vi "CAN Position Control Encoder.vi"() -> ()   [LabVIEW 2014]
doc: "This example shows how to position a motor using CAN Jaguar and a quadrature encoder. For details setting up and understanding CAN Jaguar, see the Can Jaguar Fundamentals tutorial accessable from the LabVIEW Getting Started Window.\n\nTo position the motor, a PID control loop runs on the Jaguar. Notice that the encoder is wired directly to the Jaguar. One advantage of this is that the PID control does not use resources on the roboRIO. One disadvantage is that the PID code cannot be viewed or changed. However, the control can be tuned by changing the PID Parameters.\n\nOn the diagram, notice that in order to apply new PID tuning parameters, the motor must first be disabled, and then enabled afterward. Also notice that since the control loop runs on the Jaguar, the LabVIEW loop delay is set to a slow 100ms. In fact the only reason this loop needs to run is to send a new set position, read the current position, or apply new tuning parameters.\n\nCorrect tuning parameters for a PID controller are dependent on the complete system of the motor and the load. It will be difficult to tune this system if there is no load attached to the motor. While this example is not a PID tutorial, the following information may help in understanding how to tune your PID control system.\n\nP (proportional) depends on the present error, I (integral) on the accumulation of past errors, and D (derivative) is a prediction of future errors, based on the current rate of change. The proportional parameter (P) will reduce the rise time and will reduce, but never eliminate, the steady-state error. The integral parameter (I) will eliminate the steady-state error, but may make the transient response worse. The derivative parameter (D) will increase the stability of the system, reducing the overshoot, and improving the transient response. The effects of each parameter are summarized in a table on the front panel.\n\nThis example expects a USB cable connected from your development PC to the Type B USB Jack (next to the power input) on the roboRIO.\n\nThis example requires the Driver Station to be running with Teleoperated Enabled."
uses:
  <vilib>/Rock Robotics/WPI/CAN/Jaguar/SubVIs/WPI_CANJaguar_ControlMode.ctl
  <vilib>/Rock Robotics/WPI/CAN/Jaguar/SubVIs/WPI_CANJaguar_PositionReference.ctl
  <vilib>/Rock Robotics/WPI/CAN/Jaguar/SubVIs/WPI_CANJaguar_LimitMode.ctl
  <vilib>/Rock Robotics/WPI/CAN/Jaguar/SubVIs/WPI_CANJaguar_BrakeCoastMode.ctl
  <vilib>/Rock Robotics/WPI/CAN/Jaguar/SubVIs/WPI_CANJaguar_StatusSelect.ctl
  <vilib>/Rock Robotics/WPI/MotorControl/WPI_MotorControlOpenCANJaguar.vi
panel:
  in  "PID Tuning":string[][](table)=[["Parameter", "Rise Time", "Overshoot", "Settling\nTime", "Steady State\nError"], ["P", "decrease", "increase", "small\nchange", "decrease"], ["I", "decrease", "increase", "increase", "eliminate"], ["D", "small\nchange", "decrease", "decrease", "small\nchange"]]
  out "Actual Position (revolutions)":dbl(slide) scale=-10.0..10.0
  in  "D2":dbl=15.0 caption="D"
  in  "I2":dbl=0.005 caption="I"
  in  "P2":dbl=500.0 caption="P"
  in  "apply new PID":bool
  in  "D":dbl=15.0
  in  "I":dbl=0.005
  in  "P":dbl=500.0
  in  "Set Position (revolutions)":dbl(slide) scale=-10.0..10.0
  in  "Maximum Output Voltage":dbl=12.0
  in  "Reverse Limit Position":dbl=-50.0
  in  "Forward Limit Position":dbl=50.0
  in  "Encoder Codes Per Rev":u16=1250
  in  "Device Number":u8=1
  in  "stop":bool
  # "Set these inputs before running."
  # "These can be set while running."
  # "Power\nTerminals"
  # "Motor\nTerminals"
  # "Looking at the RJ12 socket on the Jaguar, standard wire colors are shown for an inserted cable.  CAN only uses pins 3 and 4.\npin 3 (red) = CAN H\npin 4 (green) = CAN L"
  # "To roboRIO CAN terminals"
  # "Terminator plug"
  # "Black Jaguar"
  # "A"
  # "B"
  # "Index"
  # "+5V"
  # "Gnd"
  # "Encoder"
  # "white\nblack\nred\ngreen\nyellow\nblue"
  # "1   2   3   4   5   6"
  # "Runtime Tuning"
  # "PID Parameters"
  # "Initial PID Parameters"
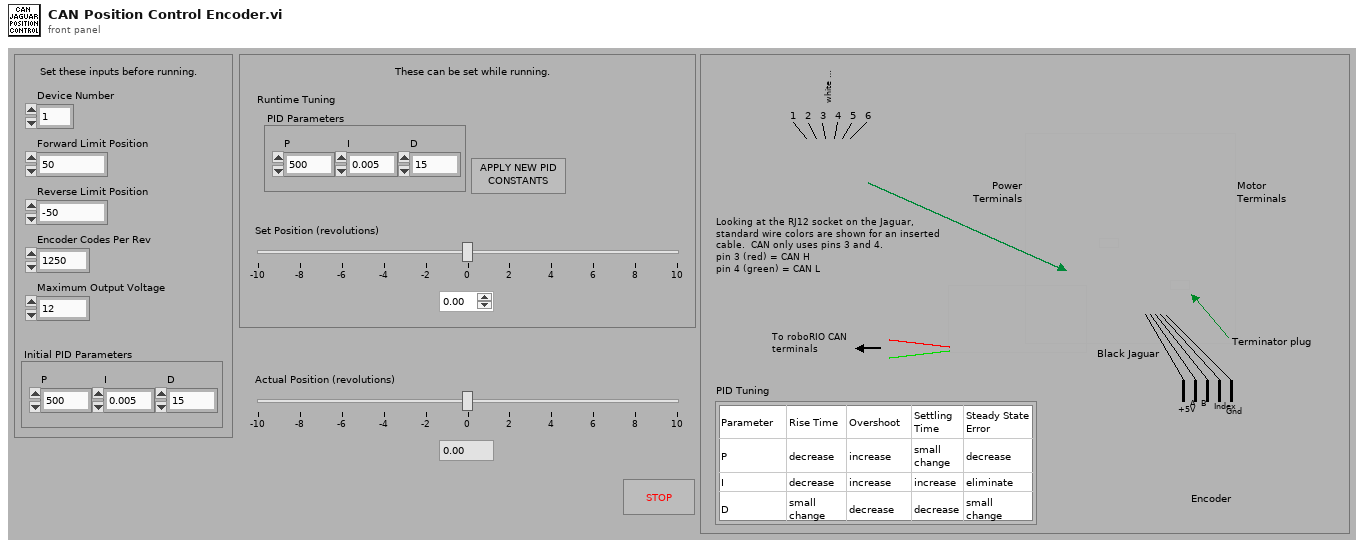
[diagram p1: front panel]
types:
  T1 = typedef "WPI_CANJaguar_StatusSelect.ctl" = enum16{"Output Percent VBus", "Output Voltage", "Bus Voltage", "Current", "Temperature", "Position", "Speed", "Limit Switches", "Faults", "Fault Counters", "Power Cycle"}
  T2 = typedef "WPI_CANJaguar_BrakeCoastMode.ctl" = enum8{"Jumper", "Brake", "Coast"}
  T3 = typedef "WPI_CANJaguar_LimitMode.ctl" = enum16{"Switch Inputs Only", "Soft Position Limits"}
  T4 = typedef "WPI_CANJaguar_PositionReference.ctl" = u8
  T5 = typedef "WPI_CANJaguar_ControlMode.ctl" = enum8{"Percent VBus", "Current", "Speed", "Position", "Voltage"}
  T6 = typedef "WPI_MotorControlDeviceRef.ctl" = cluster{"DeviceStatus":errorcluster, "Type":T7, "PWM":cluster{"Controller":T8, "PWM Channel":T9, "DeadBand":T10}, "CAN":cluster{"Device Number":u8, "Control Mode":T5, "Semaphore":T11, "Max Vout":dbl, "TalonSRX Control Mode":T12}, "Invert":bool, "TransformRef":T13, "InvTransformRef":T13}
  T7 = typedef "WPI_MotorControlType.ctl" = enum16{"PWM", "CAN", "CANTalonSRX"}
  T8 = typedef "FPGA_TypedefDigitalModule.ctl" = enum16{"Controller 1"}
  T9 = typedef "FPGA_DIOPWMChannel.ctl" = enum8{"PWM 0", "PWM 1", "PWM 2", "PWM 3", "PWM 4", "PWM 5", "PWM 6", "PWM 7", "PWM 8", "PWM 9", "PWM MXP 0", "PWM MXP 1", "PWM MXP 2", "PWM MXP 3", "PWM MXP 4", "PWM MXP 5", "PWM MXP 6", "PWM MXP 7", "PWM MXP 8", "PWM MXP 9", "Invalid"}
  T10 = typedef "WPI_PWMDeadband.ctl" = cluster{"Name":string, "maxPositivePwm":i32, "minPositivePwm":i32, "centerPwm":i32, "maxNegativePwm":i32, "minNegativePwm":i32, "angularRange":u16}
  T11 = typedef "Semaphore RefNum" = refnum<k1>
  T12 = typedef "WPI_CANTalonSRX_APIControlMode.ctl" = enum8{"Percent VBus", "Speed", "Position", "Slave", "Unchanged / Invalid"}
  T13 = typedef "WPI_PWMTransform_ConPane.ctl" = refnum<vi>
  T14 = typedef "WPI_CANJaguar_Status.ctl" = cluster{"Output Percent VBus":dbl, "Output Voltage":dbl, "Bus Voltage":dbl, "Current":dbl, "Temperature":dbl, "Position":dbl, "Speed":dbl, "Limits":cluster{"Forward Limit":bool, "Reverse Limit":bool, "Forward Soft Limit":bool, "Reverse Soft Limit":bool, "Sticky Forward Limit":bool, "Sticky Reverse Limit":bool, "Sticky Forward Soft Limit":bool, "Sticky Reverse Soft Limit":bool}, "Faults":cluster{"Current Fault":bool, "Temperature Fault":bool, "Bus Voltage Fault":bool, "Gate Driver Fault":bool, "Comm Fault":bool}, "Fault Counters":cluster{"Current Faults":u8, "Temperature Faults":u8, "Bus Voltage Faults":u8, "Gate Driver Faults":u8, "Comm Faults":u8, "CAN Status":u8, "CAN RX Errors":u8, "CAN TX Errors":u8}, "Power Cycle":bool}
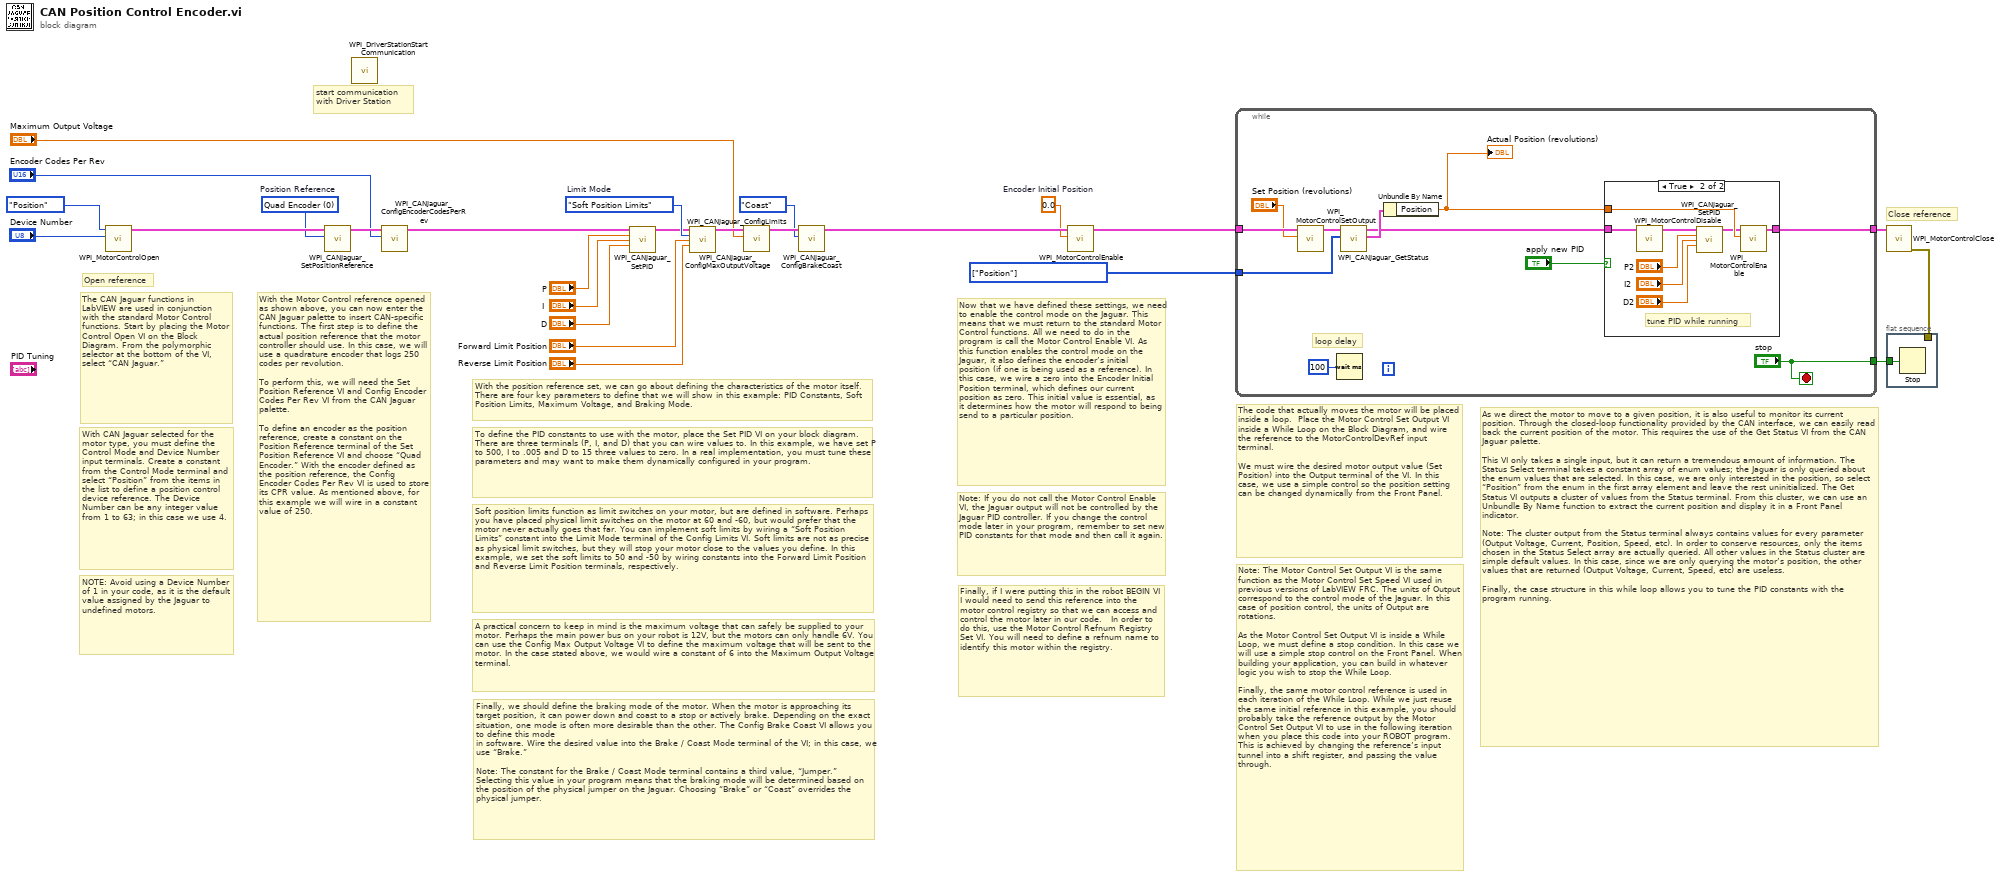
[diagram p0: block diagram]
diagram:
  w6 = 0.0  # Encoder Initial Position
  w7 = T1[] [enum."Position"] items=["Output Percent VBus", "Output Voltage", "Bus Voltage", "Current", "Temperature", "Position", "Speed", "Limit Switches", "Faults", "Fault Counters", "Power Cycle"] ("Status Select")
  w18 = WPI_CANJaguar_LimitMode."Soft Position Limits"  # Limit Mode
  w19 = T4 0 items=["Quad Encoder"=0, "Potentiometer"=1, "None"=255]  # Position Reference
  # "As we direct the motor to move to a given position, it is also useful to monitor its current position. Through the closed-loop functionality provided by the CAN interface, we can easily read back the current position of the motor. This requires the use of the Get Status VI from the CAN Jaguar palette.\n\nThis VI only takes a single input, but it can return a tremendous amount of information. The Status Select terminal takes a constant array of enum values; the Jaguar is only queried about the enum values that are selected. In this case, we are only interested in the position, so select “Position” from the enum in the first array element and leave the rest uninitialized. The Get Status VI outputs a cluster of values from the Status terminal. From this cluster, we can use an Unbundle By Name function to extract the current position and display it in a Front Panel indicator.\n\nNote: The cluster output from the Status terminal always contains values for every parameter (Output Voltage, Current, Position, Speed, etc). In order to conserve resources, only the items chosen in the Status Select array are actually queried. All other values in the Status cluster are simple default values. In this case, since we are only querying the motor’s position, the other values that are returned (Output Voltage, Current, Speed, etc) are useless.\n\nFinally, the case structure in this while loop allows you to tune the PID constants with the program running."
  # "Note: The Motor Control Set Output VI is the same function as the Motor Control Set Speed VI used in previous versions of LabVIEW FRC. The units of Output correspond to the control mode of the Jaguar. In this case of position control, the units of Output are rotations.\n\nAs the Motor Control Set Output VI is inside a While Loop, we must define a stop condition. In this case we will use a simple stop control on the Front Panel. When building your application, you can build in whatever logic you wish to stop the While Loop. \n\nFinally, the same motor control reference is used in each iteration of the While Loop. While we just reuse the same initial reference in this example, you should probably take the reference output by the Motor Control Set Output VI to use in the following iteration when you place this code into your ROBOT program. This is achieved by changing the reference’s input tunnel into a shift register, and passing the value through."
  # "The code that actually moves the motor will be placed inside a loop.  Place the Motor Control Set Output VI inside a While Loop on the Block Diagram, and wire the reference to the MotorControlDevRef input terminal. \n\nWe must wire the desired motor output value (Set Position) into the Output terminal of the VI. In this case, we use a simple control so the position setting can be changed dynamically from the Front Panel."
  # "Finally, if I were putting this in the robot BEGIN VI I would need to send this reference into the motor control registry so that we can access and control the motor later in our code.   In order to do this, use the Motor Control Refnum Registry Set VI. You will need to define a refnum name to identify this motor within the registry."
  # "Note: If you do not call the Motor Control Enable VI, the Jaguar output will not be controlled by the Jaguar PID controller. If you change the control mode later in your program, remember to set new PID constants for that mode and then call it again."
  # "Now that we have defined these settings, we need to enable the control mode on the Jaguar. This means that we must return to the standard Motor Control functions. All we need to do in the program is call the Motor Control Enable VI. As this function enables the control mode on the Jaguar, it also defines the encoder’s initial position (if one is being used as a reference). In this case, we wire a zero into the Encoder Initial Position terminal, which defines our current position as zero. This initial value is essential, as it determines how the motor will respond to being send to a particular position."
  # "Finally, we should define the braking mode of the motor. When the motor is approaching its target position, it can power down and coast to a stop or actively brake. Depending on the exact situation, one mode is often more desirable than the other. The Config Brake Coast VI allows you to define this mode\nin software. Wire the desired value into the Brake / Coast Mode terminal of the VI; in this case, we use “Brake.”\n\nNote: The constant for the Brake / Coast Mode terminal contains a third value, “Jumper.” Selecting this value in your program means that the braking mode will be determined based on the position of the physical jumper on the Jaguar. Choosing “Brake” or “Coast” overrides the physical jumper."
  # "A practical concern to keep in mind is the maximum voltage that can safely be supplied to your motor. Perhaps the main power bus on your robot is 12V, but the motors can only handle 6V. You can use the Config Max Output Voltage VI to define the maximum voltage that will be sent to the motor. In the case stated above, we would wire a constant of 6 into the Maximum Output Voltage terminal."
  # "Soft position limits function as limit switches on your motor, but are defined in software. Perhaps you have placed physical limit switches on the motor at 60 and -60, but would prefer that the motor never actually goes that far. You can implement soft limits by wiring a “Soft Position Limits” constant into the Limit Mode terminal of the Config Limits VI. Soft limits are not as precise as physical limit switches, but they will stop your motor close to the values you define. In this example, we set the soft limits to 50 and -50 by wiring constants into the Forward Limit Position and Reverse Limit Position terminals, respectively."
  # "To define the PID constants to use with the motor, place the Set PID VI on your block diagram. There are three terminals (P, I, and D) that you can wire values to. In this example, we have set P to 500, I to .005 and D to 15 three values to zero. In a real implementation, you must tune these parameters and may want to make them dynamically configured in your program."
  # "With the position reference set, we can go about defining the characteristics of the motor itself. There are four key parameters to define that we will show in this example: PID Constants, Soft Position Limits, Maximum Voltage, and Braking Mode."
  # "With the Motor Control reference opened as shown above, you can now enter the CAN Jaguar palette to insert CAN-specific functions. The first step is to define the actual position reference that the motor controller should use. In this case, we will use a quadrature encoder that logs 250 codes per revolution.\n\nTo perform this, we will need the Set Position Reference VI and Config Encoder Codes Per Rev VI from the CAN Jaguar palette. \n\nTo define an encoder as the position reference, create a constant on the Position Reference terminal of the Set Position Reference VI and choose “Quad Encoder.” With the encoder defined as the position reference, the Config Encoder Codes Per Rev VI is used to store its CPR value. As mentioned above, for this example we will wire in a constant value of 250."
  # "The CAN Jaguar functions in LabVIEW are used in conjunction with the standard Motor Control functions. Start by placing the Motor Control Open VI on the Block Diagram. From the polymorphic selector at the bottom of the VI, select “CAN Jaguar.”"
  # "NOTE: Avoid using a Device Number of 1 in your code, as it is the default value assigned by the Jaguar to undefined motors."
  # "With CAN Jaguar selected for the motor type, you must define the Control Mode and Device Number input terminals. Create a constant from the Control Mode terminal and select “Position” from the items in the list to define a position control device reference. The Device Number can be any integer value from 1 to 63; in this case we use 4."
  # "Open reference"
  # "start communication with Driver Station"
  # "Close reference"
  n1 = call-poly <vilib>:"WPI_MotorControlOpen.vi"("Device Number"="Device Number", "Control Mode"=WPI_CANJaguar_ControlMode."Position") -> ("MotorControlDeviceRef"=w23:T6)  [unwired: 4 in, 5 out]
  n2 = call <vilib>:"WPI_CANJaguar_SetPositionReference.vi"("Position Reference"=w19, "CAN Jaguar Ref"=w23) -> ("CAN Jaguar Ref Out"=w22:T6)  [unwired: 8 in, 1 out]
  n3 = call <vilib>:"WPI_DriverStationStart Communication.vi"() -> ()  [unwired: 2 in, 10 out]
  n4 = call <vilib>:"WPI_CANJaguar_ConfigEncoderCodesPerRev.vi"("Encoder Codes Per Rev"="Encoder Codes Per Rev", "CAN Jaguar Ref"=w22) -> ("CAN Jaguar Ref Out"=w21:T6)  [unwired: 8 in, 1 out]
  n5 = call <vilib>:"WPI_CANJaguar_SetPID.vi"("CAN Jaguar Ref"=w21, "P"="P", "I"="I", "D"="D") -> ("CAN Jaguar Ref Out"=w10:T6)  [unwired: 10 in, 1 out]
  n6 = call <vilib>:"WPI_CANJaguar_ConfigLimits.vi"("CAN Jaguar Ref"=w10, "Limit Mode"=w18, "Forward Limit Position"="Forward Limit Position", "Reverse Limit Position"="Reverse Limit Position") -> ("CAN Jaguar Ref Out"=w14:T6)  [unwired: 10 in, 1 out]
  n7 = call <vilib>:"WPI_CANJaguar_ConfigMaxOutputVoltage.vi"("Maximum Output Voltage"="Maximum Output Voltage", "CAN Jaguar Ref"=w14) -> ("CAN Jaguar Ref Out"=w15:T6)  [unwired: 8 in, 1 out]
  n8 = call <vilib>:"WPI_CANJaguar_ConfigBrakeCoast.vi"("Brake / Coast Mode"=WPI_CANJaguar_BrakeCoastMode."Coast", "CAN Jaguar Ref"=w15) -> ("CAN Jaguar Ref Out"=w11:T6)  [unwired: 8 in, 1 out]
  n9 = call <vilib>:"WPI_MotorControlEnable.vi"("Encoder Initial Position"=w6, "CAN Jaguar Ref"=w11) -> ("CAN Jaguar Ref Out"=w9:T6)  [unwired: 8 in, 1 out]
  n10 = while {
    tunnel: ["stop"] -> w2
    tunnel: w9 -> [w34]
    tunnel: [w29] -> w8
    tunnel: w7 -> [w32]
    stop <- "stop" stop-if-true
    # "loop delay"
    n11 = call <vilib>:"WPI_MotorControlSetOutput.vi"("Output"="Set Position (revolutions)", "MotorControlDevRef"=w34) -> ("MotorControlDevRef"=w33:T6)  [unwired: 7 in, 2 out]
    n12 = Wait (ms)(milliseconds to wait=u32 100) -> ()  [unwired: 1 out]
    n13 = call <vilib>:"WPI_CANJaguar_GetStatus.vi"("Status Select"=w32, "CAN Jaguar Ref"=w33) -> ("Status"=w31:T14, "CAN Jaguar Ref Out"=w30:T6)  [unwired: 7 in, 1 out]
    n14 = Unbundle By Name(w31) -> ("Position"=w26:dbl)
    "Actual Position (revolutions)" <- w26
    n15 = case shown="True" "apply new PID" {
      tunnel: w30 -> [w37 w42]
      tunnel: w26 -> [_ w45]
      tunnel: [w37 w43] -> w29
      frame False {
      }
      frame True {
        # "tune PID while running"
        n16 = call <vilib>:"WPI_MotorControlDisable.vi"("MotorControlDevRef"=w42) -> ("MotorControlDevRef"=w41:T6)  [unwired: 9 in, 1 out]
        n17 = call <vilib>:"WPI_CANJaguar_SetPID.vi"("CAN Jaguar Ref"=w41, "P"="P2", "I"="I2", "D"="D2") -> ("CAN Jaguar Ref Out"=w44:T6)  [unwired: 10 in, 1 out]
        n18 = call <vilib>:"WPI_MotorControlEnable.vi"("Encoder Initial Position"=w45, "CAN Jaguar Ref"=w44) -> ("CAN Jaguar Ref Out"=w43:T6)  [unwired: 8 in, 1 out]
      }
    }
  }
  n19 = call <vilib>:"WPI_MotorControlClose.vi"("MotorControlDevRef"=w8) -> ("error out"=w1:errorcluster)  [unwired: 10 in]
  n20 = flat-sequence {
    tunnel: w2 -> [w46]
    tunnel: w1 -> [_]
    frame #0 {
      n21 = Stop(stop? (T)=w46) -> ()
    }
  }
